vi "Run.vi"(8 "error in (no error)":errorcluster, 11 "Channel Sub in":refnum<class "Channel Sub.lvclass">) -> (0 "error out":errorcluster, 3 "Channel Sub out":refnum<class "Channel Sub.lvclass">)   [LabVIEW 2018, in "Channel Sub.lvclass"]
uses:
  Channel Sub.lvclass
  Communication Channel/Communication Channel.lvclass
  State Machine/State Machine.lvclass
  RxTx/RxTx.lvclass
  Socket/Socket.lvclass
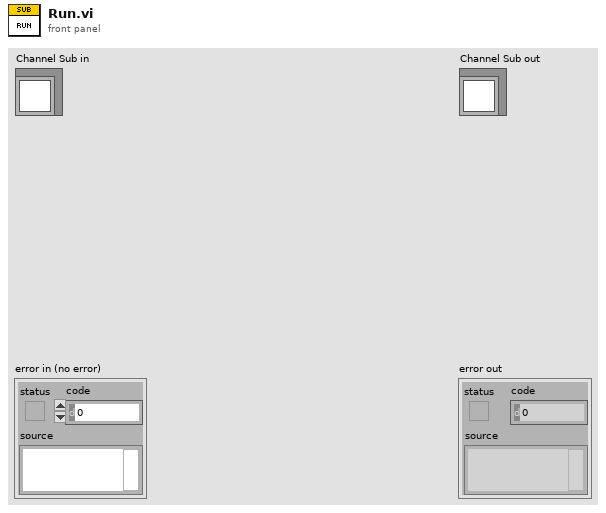
[diagram p1: front panel]
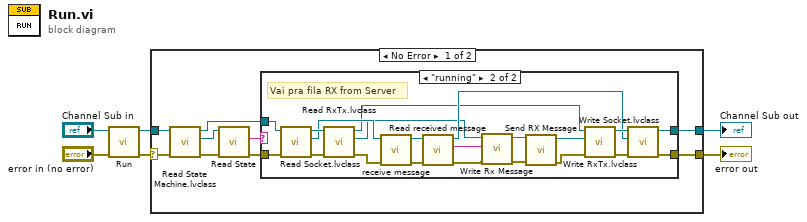
[diagram p0: block diagram]
diagram:
  n1 = call-parent "Run.vi"("error in (no error)"="error in (no error)", "Communication Channel in"="Channel Sub in") -> ("error out"=w3:errorcluster, "Communication Channel out"=w4:refnum<class "Channel Sub.lvclass">)  [unwired: 8 in]
  n2 = case shown="No Error" w3 {
    selector: w3 -> [w14 w39]
    tunnel: w4 -> [w15 w40]
    tunnel: [w8 w40] -> w2
    tunnel: [w9 w39] -> w1
    frame No Error {
      n3 = call-dynamic "Read State Machine.lvclass.vi"("error in (no error)"=w14, "Communication Channel in"=w15) -> ("error out"=w13:errorcluster, "State Machine.lvclass"=w10:refnum<class "State Machine.lvclass">, "Communication Channel out"=w11:refnum<class "Channel Sub.lvclass">)  [unwired: 7 in]
      n4 = call-dynamic "Read State.vi"("error in (no error)"=w13, "State Machine in"=w10) -> ("error out"=w7:errorcluster, "State"=w12:string)  [unwired: 7 in, 1 out]
      n5 = case shown="\"running\"" w12 {
        tunnel: w11 -> [w17 w38]
        tunnel: [w17 w34] -> w8
        tunnel: [w16 w32] -> w9
        tunnel: w7 -> [w16 w31]
        frame Default {
        }
        frame "running" {
          # "Vai pra fila RX from Server"
          n6 = call-dynamic "Read Socket.lvclass.vi"("error in (no error)"=w31, "Communication Channel in"=w38) -> ("error out"=w36:errorcluster, "Socket.lvclass"=w28:refnum<class "Socket.lvclass">, "Communication Channel out"=w37:refnum<class "Channel Sub.lvclass">)  [unwired: 7 in]
          n7 = call-dynamic "Read RxTx.lvclass.vi"("error in (no error)"=w36, "Communication Channel in"=w37) -> ("error out"=w24:errorcluster, "RxTx.lvclass"=w22:refnum<class "RxTx.lvclass">, "Communication Channel out"=w25:refnum<class "Channel Sub.lvclass">)  [unwired: 7 in]
          n8 = call-dynamic "receive message.vi"("error in (no error)"=w24, "Socket in"=w28) -> ("error out"=w30:errorcluster, "Socket out"=w29:refnum<class "Socket.lvclass">)  [unwired: 8 in]
          n9 = call-dynamic "Read received message.vi"("error in (no error)"=w30, "Socket in"=w29) -> ("error out"=w19:errorcluster, "received message"=w20:string, "Socket out"=w27:refnum<class "Socket.lvclass">)  [unwired: 7 in]
          n10 = call "Write Rx Message.vi"("error in (no error)"=w19, "Rx Message"=w20, "RxTx in"=w22) -> ("error out"=w18:errorcluster, "RxTx out"=w21:refnum<class "RxTx.lvclass">)  [unwired: 7 in]
          n11 = call "Send RX Message.vi"("error in (no error)"=w18, "RxTx in"=w21) -> ("error out"=w23:errorcluster, "RxTx out"=w26:refnum<class "RxTx.lvclass">)  [unwired: 8 in]
          n12 = call-dynamic "Write RxTx.lvclass.vi"("error in (no error)"=w23, "RxTx.lvclass"=w26, "Communication Channel in"=w25) -> ("error out"=w33:errorcluster, "Communication Channel out"=w35:refnum<class "Channel Sub.lvclass">)  [unwired: 7 in]
          n13 = call-dynamic "Write Socket.lvclass.vi"("error in (no error)"=w33, "Socket2.lvclass"=w27, "Communication Channel in"=w35) -> ("error out"=w32:errorcluster, "Communication Channel out"=w34:refnum<class "Channel Sub.lvclass">)  [unwired: 7 in]
        }
      }
    }
    frame Error {
    }
  }
  "error out" <- w1
  "Channel Sub out" <- w2
